vi "Query Phase Noise Marker.vi"(0 "VISA resource name":refnum<visa-resource-name>, 7 "Select Marker (1: Marker 1)":i32(ring)=1 items=["Marker 1"=1, "Marker 2"=2, "Marker 3"=3, "Marker 4"=4], 11 "error in (no error)":errorcluster) -> (4 "VISA resource name out":refnum<visa-resource-name>, 6 "Marker X-Axis Position":dbl, 8 "Marker Y-Axis Position":dbl, 15 "error out":errorcluster)   [LabVIEW 2014, in "Agilent ESA PSA Series.lvlib"]
doc: "Returns the marker operation results for the Log Plot measurement of the Phase Noise personality.\n\n<B>Note:</B> \n\nThis VI is only valid in Phase Noise personality. Use <B>Switch Personality</B> VI to switch to Phase Noise before calling this VI."
uses:
  Agilent ESA PSA Series.lvlib
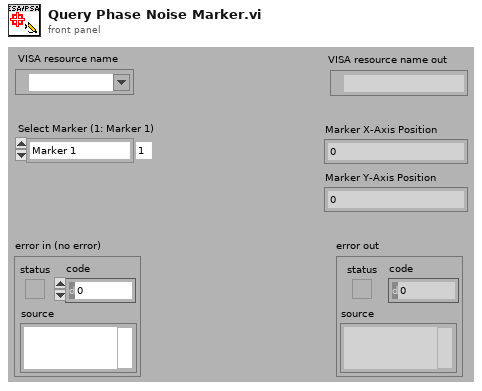
[diagram p1: front panel]
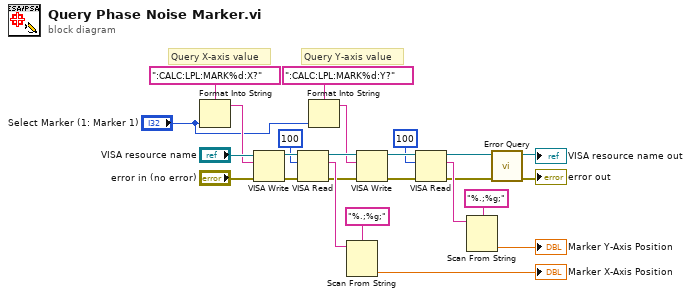
[diagram p0: block diagram]
diagram:
  # "Query Y-axis value"
  # "Query X-axis value"
  n1 = Format Into String(format string=":CALC:LPL:MARK%d:X?", "Select Marker (1: Marker 1)") -> (resulting string=w20:string)  [unwired: 2 in, 1 out]
  n2 = VISA Write(VISA resource name="VISA resource name", write buffer=w20, error in (no error)="error in (no error)") -> (VISA resource name out=w19:refnum<visa-resource-name>, error out=w18:errorcluster)  [unwired: 1 out]
  n3 = VISA Read(VISA resource name=w19, byte count=u32 100, error in (no error)=w18) -> (VISA resource name out=w15:refnum<visa-resource-name>, read buffer=w17:string, error out=w14:errorcluster)  [unwired: 1 out]
  n4 = Format Into String(format string=":CALC:LPL:MARK%d:Y?", "Select Marker (1: Marker 1)") -> (resulting string=w11:string)  [unwired: 2 in, 1 out]
  n5 = Scan From String(format string="%.;%g;", input string=w17) -> (output 1=→"Marker X-Axis Position":dbl)  [unwired: 3 in, 3 out]
  n6 = VISA Write(VISA resource name=w15, write buffer=w11, error in (no error)=w14) -> (VISA resource name out=w9:refnum<visa-resource-name>, error out=w10:errorcluster)  [unwired: 1 out]
  n7 = VISA Read(VISA resource name=w9, byte count=u32 100, error in (no error)=w10) -> (VISA resource name out=w3:refnum<visa-resource-name>, read buffer=w7:string, error out=w4:errorcluster)  [unwired: 1 out]
  n8 = Scan From String(format string="%.;%g;", input string=w7) -> (output 1=→"Marker Y-Axis Position":dbl)  [unwired: 3 in, 3 out]
  n9 = call "Error Query.vi"("error in (no error)"=w4, "VISA resource name"=w3) -> ("error out"=→"error out":errorcluster, "VISA resource name out"=→"VISA resource name out":refnum<visa-resource-name>)  [unwired: 6 in, 2 out]
